vi "Teleop_Calc_Flywheel.vi"(11 "Teleop Local Data in":T1) -> (3 "Teleop Local Data out":T1)   [LabVIEW 2016]
uses:
  Typedefs/typedef_cluster_Teleop Local Data.ctl
  Typedefs/typedef_enum_Joystick Buttons.ctl
panel:
  out "Sensor RPM":dbl
  in  "Low Goal":dbl(slide)=2200.0 scale=2000.0..4000.0
  in  "High Goal":dbl(slide)=3200.0 scale=2000.0..4000.0
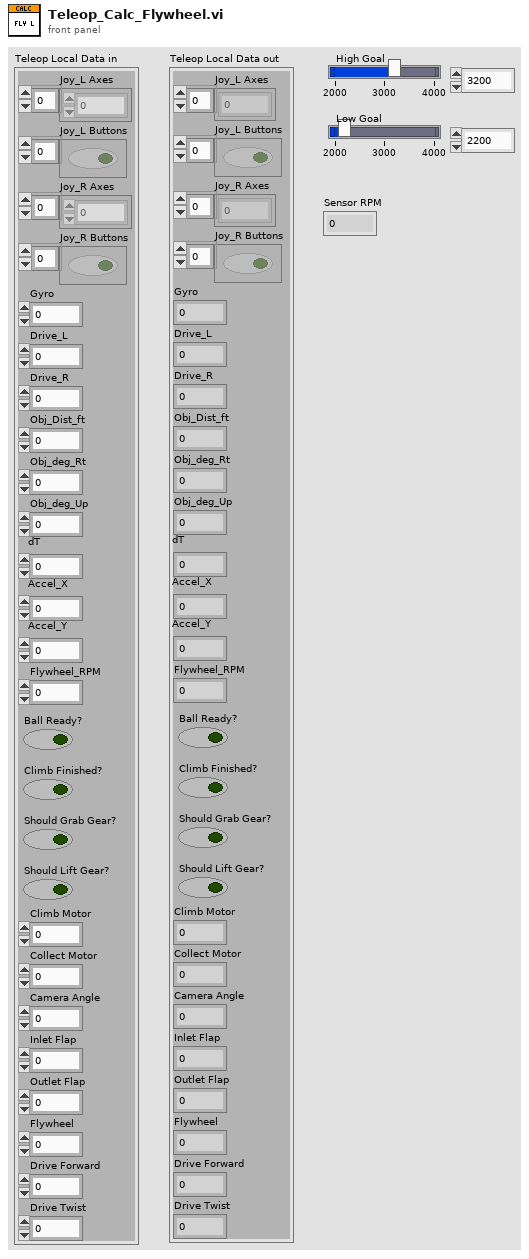
[diagram p1: front panel]
types:
  T1 = typedef "typedef_cluster_Teleop Local Data.ctl" = cluster{"Joy_L Axes":dbl[], "Joy_L Buttons":bool[], "Joy_R Axes":dbl[], "Joy_R Buttons":bool[], "Gyro":dbl, "Drive_L":i32, "Drive_R":i32, "Obj_Dist_ft":dbl, "Obj_deg_Rt":dbl, "Obj_deg_Up":dbl, "dT":dbl, "Accel_X":dbl, "Accel_Y":dbl, "Flywheel_RPM":dbl, "Ball Ready?":bool, "Climb Finished?":bool, "Should Grab Gear?":bool, "Should Lift Gear?":bool, "Climb Motor":dbl, "Collect Motor":dbl, "Camera Angle":dbl, "Inlet Flap":dbl, "Outlet Flap":dbl, "Flywheel":dbl, "Drive Forward":dbl, "Drive Twist":dbl}
  T2 = typedef "typedef_enum_Joystick Buttons.ctl" = enum16{"Trigger", "Thumb", "Top3", "Top4", "Top5", "Top6", "Low7", "Low8", "Low9", "Low10", "Low11", "Low12", "Hat0", "Hat1", "Hat2", "Hat3", "Hat4", "Hat5", "Hat6", "Hat7", "Hat8"}
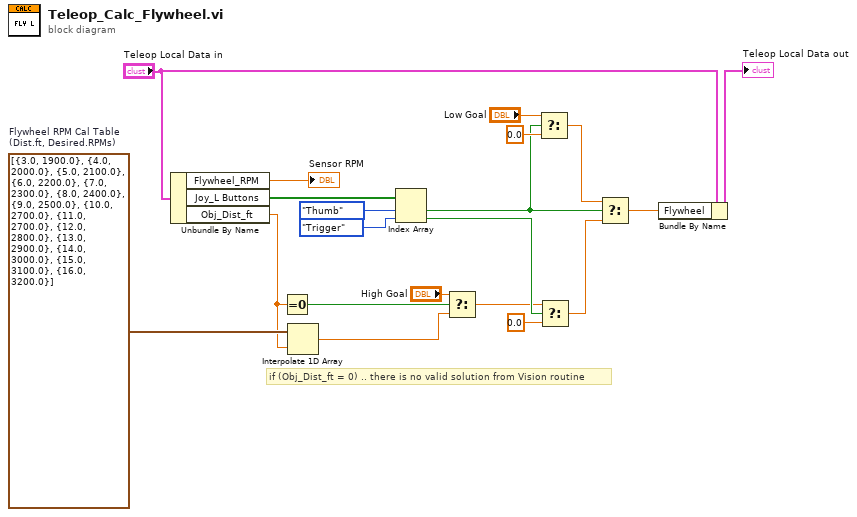
[diagram p0: block diagram]
diagram:
  w9 = cluster{dbl, dbl}[] [{3.0, 1900.0}, {4.0, 2000.0}, {5.0, 2100.0}, {6.0, 2200.0}, {7.0, 2300.0}, {8.0, 2400.0}, {9.0, 2500.0}, {10.0, 2700.0}, {11.0, 2700.0}, {12.0, 2800.0}, {13.0, 2900.0}, {14.0, 3000.0}, {15.0, 3100.0}, {16.0, 3200.0}]  # Flywheel RPM Cal Table (Dist.ft, Desired.RPMs)
  # "if (Obj_Dist_ft = 0) .. there is no valid solution from Vision routine"
  n1 = Unbundle By Name("Teleop Local Data in") -> ("Flywheel_RPM"=→"Sensor RPM":dbl, "Joy_L Buttons"=w18:bool[], "Obj_Dist_ft"=w8:dbl)
  n2 = Equal To 0?(x=w8) -> (x = 0?=w3:bool)
  n3 = Interpolate 1D Array(1:w8, 2:w9) -> (0:w2:dbl)
  n4 = Index Array(array=w18, index #1=typedef_enum_Joystick_Buttons."Thumb" ("Joystick Buttons"), index #2=typedef_enum_Joystick_Buttons."Trigger" ("Joystick Buttons")) -> (element #1=w6:bool, element #2=w16:bool)
  n5 = Select(t="High Goal", s=w3, f=w2) -> (s? t:f=w4:dbl)
  n6 = Select(t="Low Goal", s=w6, f=0.0) -> (s? t:f=w12:dbl)
  n7 = Select(t=w4, s=w16, f=0.0) -> (s? t:f=w11:dbl)
  n8 = Select(t=w12, s=w6, f=w11) -> (s? t:f=w10:dbl)
  n9 = Bundle By Name(cluster="Teleop Local Data in", "Flywheel"=w10) -> (→"Teleop Local Data out":T1)
